vi "Color_select_for_LED.vi"() -> (2 "Array":u32[](array[numeric]), 3 "Boolean":bool)   [LabVIEW 2020]
uses:
  <vilib>/Rock Robotics/WPI/DriverStation/WPI_DriverStationRobotMode2.ctl
  Robot Global Data.vi
  Globals/Climber_Globals.vi
  Globals/Flywheel_Globals.vi
  Globals/Turret_Globals.vi
  Globals/Cowl_Globals.vi
  Globals/Sensor_Values.vi
  Globals/Autonomous_Globals.vi
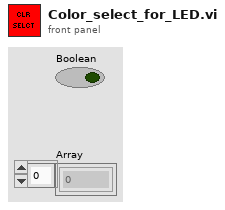
[diagram p1: front panel]
types:
  T1 = typedef "WPI_DriverStationRobotMode2.ctl" = enum16{"Autonomous Disabled", "Autonomous Enabled", "Teleop Disabled", "Teleop Enabled", "Disconnected", "Finish", "Test Disabled", "Test Enabled", "Emergency Stopped"}
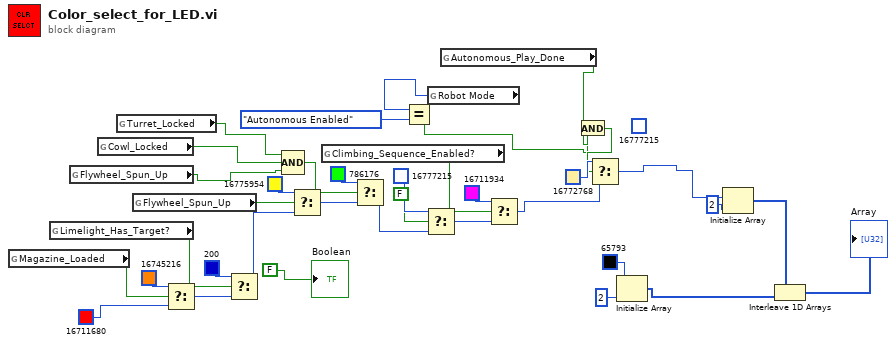
[diagram p0: block diagram]
diagram:
  (unwired) u32 16777215
  n1 = global read "Sensor_Values.vi" "Magazine_Loaded"() -> (w27:bool)
  n2 = global read "Sensor_Values.vi" "Limelight_Has_Target?"() -> (w26:bool)
  n3 = global read "Flywheel_Globals.vi" "Flywheel_Spun_Up"() -> (w35:bool)
  n4 = global read "Cowl_Globals.vi" "Cowl_Locked"() -> (w34:bool)
  n5 = global read "Turret_Globals.vi" "Turret_Locked"() -> (w33:bool)
  n6 = global read "Flywheel_Globals.vi" "Flywheel_Spun_Up"() -> (w17:bool)
  n7 = Select(t=u32 16745216, s=w27, f=u32 16711680) -> (s? t:f=w18:u32)
  n8 = Select(t=u32 200, s=w26, f=w18) -> (s? t:f=w19:u32)
  n9 = Compound Arithmetic op=AND(w33, w34, w35) -> (w16:bool)
  n10 = Select(t=u32 16775954, s=w17, f=w19) -> (s? t:f=w11:u32)
  n11 = global read "Climber_Globals.vi" "Climbing_Sequence_Enabled?"() -> (w14:bool)
  n12 = Select(t=u32 786176, s=w16, f=w11) -> (s? t:f=w8:u32)
  n13 = Select(t=u32 16777215, s=FALSE, f=w8) -> (s? t:f=w9:u32)
  n14 = global read "Robot Global Data.vi" "Robot Mode"() -> (w12:T1)
  n15 = Equal?(x=w12, y=WPI_DriverStationRobotMode2."Autonomous Enabled") -> (x = y?=w28:bool)
  n16 = global read "Autonomous_Globals.vi" "Autonomous_Play_Done"() -> (w29:bool)
  n17 = Select(t=u32 16711934, s=w14, f=w9) -> (s? t:f=w10:u32)
  n18 = And(x=w29, y=w28) -> (x .and. y?=w30:bool)
  n19 = Select(t=u32 16772768, s=w30, f=w10) -> (s? t:f=w1:u32)
  n20 = Initialize Array(u32 65793, 2 ("dimension size")) -> (w3:u32[])
  n21 = Initialize Array(w1, 2 ("dimension size")) -> (w5:u32[])
  n22 = Interleave 1D Arrays(w5, w3) -> (→"Array":u32[])
  "Boolean" <- FALSE
